vi "Get Version.vi"(8 "error in (no error)":errorcluster, 11 "DSF Buffer Converter Configurations in":refnum<class "Default Buffer Converter Configurations.lvclass">) -> (0 "error out":errorcluster, 2 "version":T1, 3 "DSF Buffer Converter Configurations out":refnum<class "Default Buffer Converter Configurations.lvclass">)   [LabVIEW 2019, in "DSF Core.lvlib" / "Default Buffer Converter Configurations.lvclass"]
uses:
  Default Buffer Converter Configurations.lvclass
  Typedefs/DSF Version Info.ctl
  DSF Core.lvlib
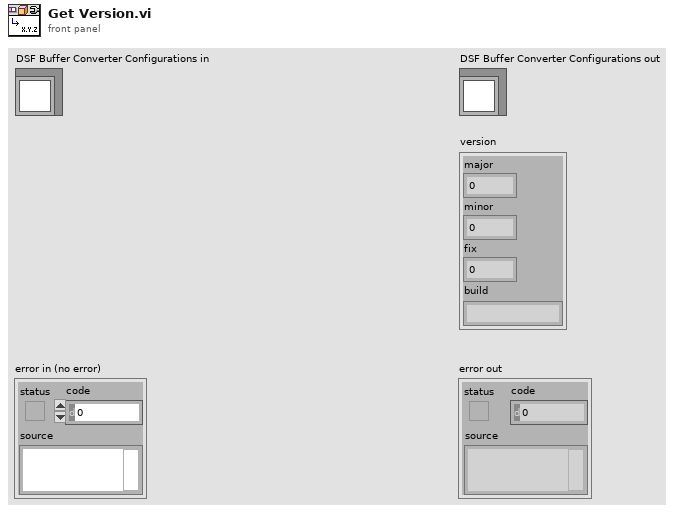
[diagram p1: front panel]
types:
  T1 = typedef "DSF Core.lvlib/DSF Version Info.ctl" = cluster{"major":u32, "minor":u32, "fix":u32, "build":string}
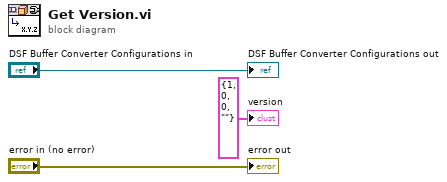
[diagram p0: block diagram]
diagram:
  "error out" <- "error in (no error)"
  "DSF Buffer Converter Configurations out" <- "DSF Buffer Converter Configurations in"
  "version" <- T1 {"major"=1, "minor"=0, "fix"=0, "build"=""} ("version")
